vi "Yscaling.vi"(7 "Nano Z Read (m)":dbl, 8 "Current Maxed?":bool, 9 "Y":dbl, 10 "Plane Height":dbl) -> (0 "y scaled (nm)":dbl, 3 "Nano Z Write (m)":dbl)   [LabVIEW 2019]
uses:
  <userlib>/HapticSTM/HapticSTM.lvlib
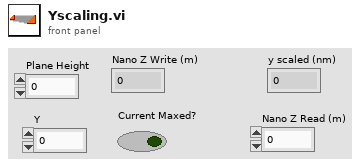
[diagram p1: front panel]
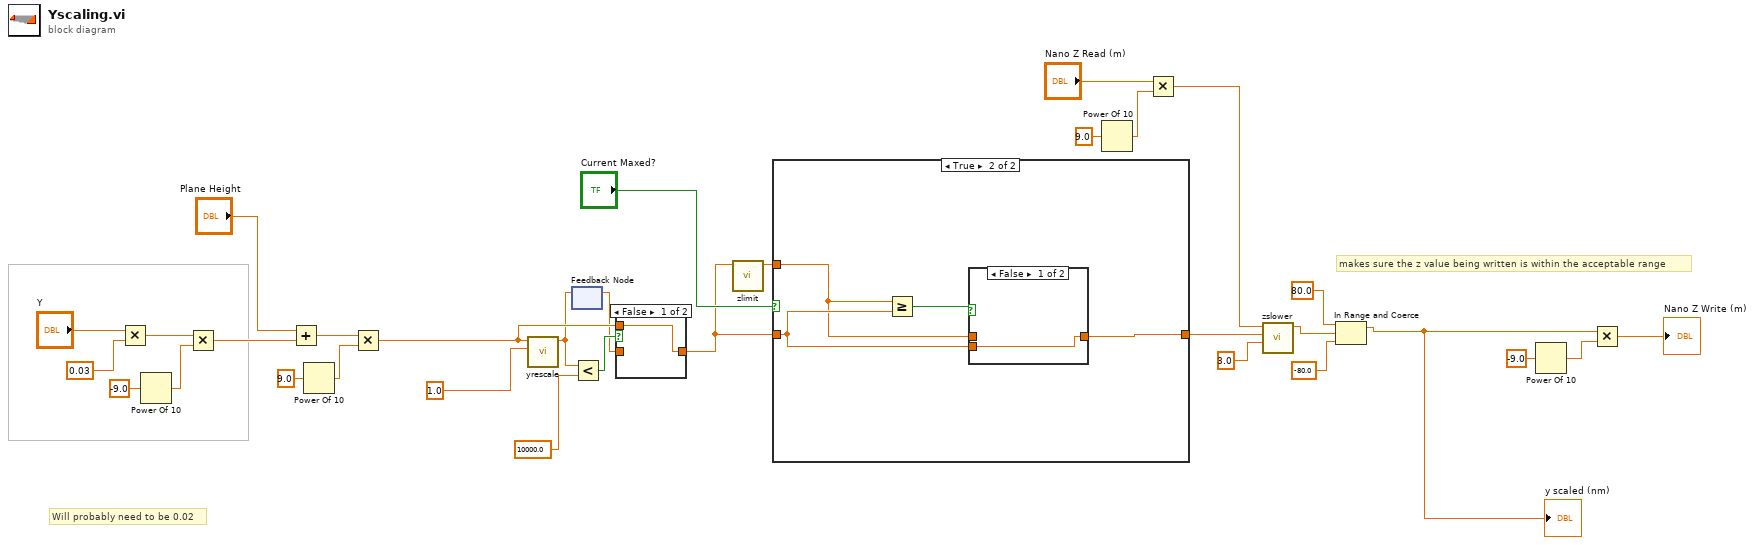
[diagram p0: block diagram]
diagram:
  # "Will probably need to be 0.02"
  # "makes sure the z value being written is within the acceptable range"
  n1 = Multiply(x="Y", y=0.03) -> (x*y=w28:dbl)
  n2 = Power Of 10(x=-9.0) -> (10^x=w27:dbl)
  n3 = Multiply(x=w28, y=w27) -> (x*y=w29:dbl)
  n4 = Add(x="Plane Height", y=w29) -> (x+y=w32:dbl)
  n5 = Power Of 10(x=9.0) -> (10^x=w31:dbl)
  n6 = Multiply(x=w32, y=w31) -> (x*y=w13:dbl)
  n7 = call <userlib>:"yrescale.vi"("scalingfactor"=1.0, "ylabview"=w13) -> ("function return"=w12:dbl)  [unwired: 9 in]
  n8 = feedback-in #1(w12) -> ()
  n9 = feedback #1() -> (w11:dbl)  [unwired: 1 in]
  n10 = Less?(x=w12, y=10000.0) -> (x < y?=w14:bool)
  n11 = case shown="False" w14 {
    tunnel: [w33 w34] -> w16
    tunnel: w11 -> [_ w34]
    tunnel: w13 -> [w33 _]
    frame False {
    }
    frame True {
    }
  }
  n12 = call <userlib>:"zlimit.vi"("yscaledinput"=w16) -> ("function return"=w17:dbl)  [unwired: 10 in]
  n13 = case shown="True" "Current Maxed?" {
    tunnel: [w35 w39] -> w10
    tunnel: w16 -> [w35 w37]
    tunnel: w17 -> [_ w36]
    frame False {
    }
    frame True {
      n14 = Greater Or Equal?(x=w36, y=w37) -> (x >= y?=w38:bool)
      n15 = case shown="False" w38 {
        tunnel: w36 -> [_ w41]
        tunnel: [w40 w41] -> w39
        tunnel: w37 -> [w40 _]
        frame False {
        }
        frame True {
        }
      }
    }
  }
  n16 = Power Of 10(x=9.0) -> (10^x=w8:dbl)
  n17 = Multiply(x="Nano Z Read (m)", y=w8) -> (x*y=w5:dbl)
  n18 = call <userlib>:"zslower.vi"("maxvel"=3.0, "labview_zpos_write"=w10, "nanonis_zpos_read"=w5) -> ("function return"=w4:dbl)  [unwired: 8 in]
  n19 = In Range and Coerce(upper limit=80.0, x=w4, lower limit=-80.0) -> (coerced(x)=w1:dbl)  [unwired: 1 out]
  "y scaled (nm)" <- w1
  n20 = Power Of 10(x=-9.0) -> (10^x=w20:dbl)
  n21 = Multiply(x=w1, y=w20) -> (x*y=→"Nano Z Write (m)":dbl)
